vi "Open.vi"(8 "error in":errorcluster, 9 "parameters":variant, 10 "file path":path, 11 "repository in":refnum<class "NISE_CEF_HierarchyRepo.lvclass">) -> (0 "error out":errorcluster, 2 "invalid?":bool, 3 "repository out":refnum<class "NISE_CEF_HierarchyRepo.lvclass">)   [LabVIEW 2013, in "NISE_CEF_HierarchyRepo.lvclass"]
doc: "Loads the saved information of the repo. It could load multiple files at the same time. An option to add file versioning could be included in the files, and the code to manage changes would be in this VI."
uses:
  NISE_CEF_HierarchyRepo.lvclass
  NISE_CEF_HierarchyRepo.lvclass/NISE_CEF_HierarchyRepo.ctl
  tree serializer/NISE_CEF_TreeSerializer.lvlib
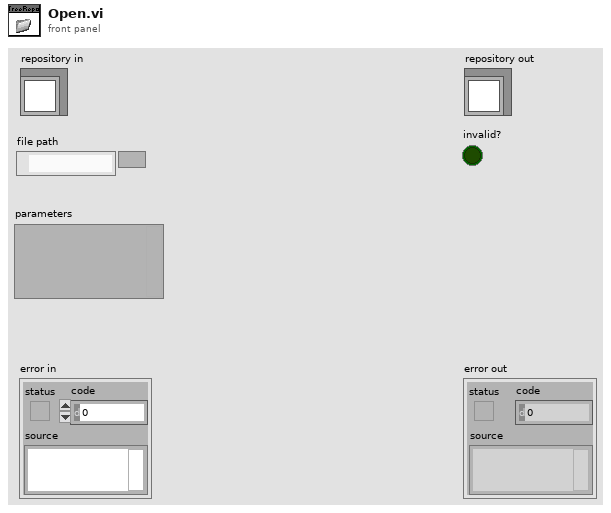
[diagram p1: front panel]
types:
  T1 = typedef "NISE_CEF_TreeSerializer.lvlib/base file format.ctl" = cluster{"version":string, "data":string}
  T2 = typedef "NISE_CEF_TreeSerializer.lvlib/file data format.ctl" = cluster{"root":string, "hierarchy":T3[], "instance data":T4[]}
  T3 = typedef "NISE_CEF_TreeSerializer.lvlib/hierarchy element.ctl" = cluster{"current node":string, "children":string[]}
  T4 = typedef "NISE_CEF_TreeSerializer.lvlib/instance data.ctl" = cluster{"ID":string, "Alias":string, "class":string, "version":string, "data":string}
  T5 = typedef "NISE_CEF_TreeSerializer.lvlib/memory hierarchy.ctl" = cluster{"root":string, "hierarchy":T3[], "instance data":refnum<class "NISE_CEF_serializable configuration.lvclass">[]}
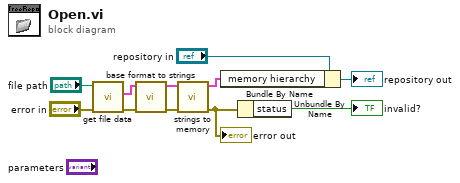
[diagram p0: block diagram]
diagram:
  n1 = call "get file data.vi"("error in"="error in", "Path"="file path") -> ("error out"=w6:errorcluster, "format"=w7:T1)  [unwired: 8 in]
  n2 = call "base format to strings.vi"("error in"=w6, "format"=w7) -> ("error out"=w5:errorcluster, "data"=w4:T2)  [unwired: 8 in]
  n3 = call "strings to memory.vi"("error in"=w5, "1.0.0"=w4) -> ("error out"=w2:errorcluster, "memory hierarchy"=w3:T5)  [unwired: 8 in]
  "error out" <- w2
  n4 = Bundle By Name(cluster="repository in", "memory hierarchy"=w3) -> (→"repository out":refnum<class "NISE_CEF_HierarchyRepo.lvclass">)
  n5 = Unbundle By Name(w2) -> ("status"=→"invalid?":bool)
